vi "Simplify File Path.vi"(8 "error in (no error)":errorcluster, 11 "full path":path) -> (0 "error out":errorcluster, 3 "simplified path":string)   [LabVIEW 2017]
doc: "Simplifies <b>full path</b> in the following way:\n• If the full path points to the LabVIEW directory, the simplified path will be [LabVIEW]\\some_folders_if_exist\\error_list.txt.\n• In other cases the simplified path will be [User]\\error_list.txt."
uses:
  <vilib>/regexp/Match Regular Expression.xnode
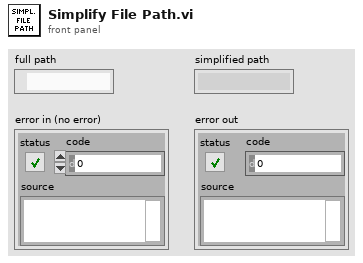
[diagram p1: front panel]
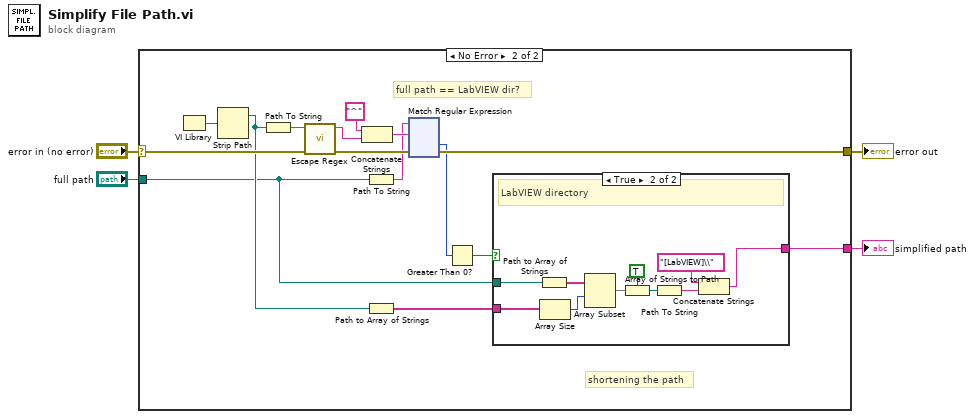
[diagram p0: block diagram]
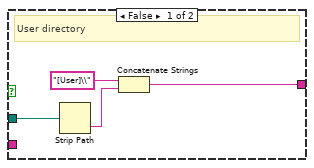
[diagram p3: hidden frame]
diagram:
  n1 = case shown="No Error" "error in (no error)" {
    selector: "error in (no error)" -> [w5 w19]
    tunnel: "full path" -> [_ w8]
    tunnel: [w5 w18] -> w2
    tunnel: [_ w6] -> w1
    frame Error {
    }
    frame No Error {
      # "shortening the path"
      # "full path == LabVIEW dir?"
      n2 = VI Library() -> (path=w11:path)
      n3 = Strip Path(path=w11) -> (stripped path=w10:path)  [unwired: 1 out]
      n4 = Path To String(path=w10) -> (string=w17:string)
      n5 = call "Escape Regex.vi"("error in (no error)"=w19, "regex"=w17) -> ("error out"=w20:errorcluster, "escaped regex"=w16:string)  [unwired: 8 in]
      n6 = Concatenate Strings("^" ("string"), w16) -> (w14:string)
      n7 = Path To String(path=w8) -> (string=w13:string)
      n8 = Path to Array of Strings(0:w10) -> (2:w7:string[])  [unwired: 1 out]
      n9 = xnode "Match Regular Expression"("input string"=w13, "regular expression"=w14, "error in"=w20) -> ("offset past match"=w12:i32, "error out"=w18:errorcluster)  [unwired: 3 in, 3 out]
      n10 = Greater Than 0?(x=w12) -> (x > 0?=w9:bool)
      n11 = case shown="True" w9 {
        tunnel: w8 -> [w22 w27]
        tunnel: w7 -> [_ w26]
        tunnel: [w21 w25] -> w6
        frame False {
          # "User directory"
          n12 = Strip Path(path=w22) -> (name=w24:string)  [unwired: 1 out]
          n13 = Concatenate Strings("[User]\\" ("string"), w24) -> (w21:string)
        }
        frame True {
          # "LabVIEW directory"
          n14 = Path to Array of Strings(0:w27) -> (2:w28:string[])  [unwired: 1 out]
          n15 = Array Size(array=w26) -> (size(s)=w34:i32)
          n16 = Array Subset(array=w28, index=w34) -> (w29:string[])  [unwired: 1 in]
          n17 = Array of Strings to Path(0:w29, 1:TRUE ("relative")) -> (2:w31:path)
          n18 = Path To String(path=w31) -> (string=w33:string)
          n19 = Concatenate Strings("[LabVIEW]\\" ("string"), w33) -> (w25:string)
        }
      }
    }
  }
  "simplified path" <- w1
  "error out" <- w2
